vi "enthalpy of vaporization.vi"(8 "error in (no error)":errorcluster, 11 "TK":dbl) -> (0 "error out":errorcluster, 3 "function return":dbl)   [LabVIEW 2011, in "fsteam.lvlib"]
doc: "extern double enthalpy_of_vaporization(double TK);"
uses:
  <userlib>/fsteam/fsteam.lvlib
  <userlib>/fsteam/fsteam.dll
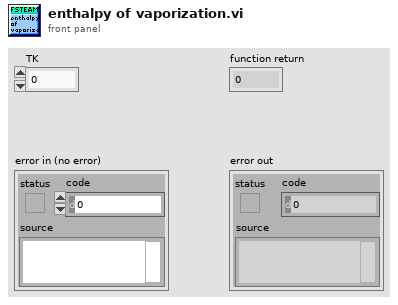
[diagram p1: front panel]
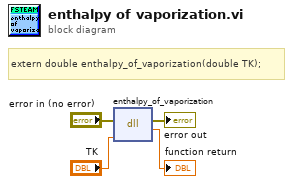
[diagram p0: block diagram]
diagram:
  # "extern double enthalpy_of_vaporization(double TK);"
  n1 = dll-call lib="C:/Program Files (x86)/National Instruments/LabVIEW 2011/user.lib/fsteam/fsteam.*" fn="enthalpy_of_vaporization"(error in="error in (no error)", "TK"="TK") -> (error out=→"error out":errorcluster, →"function return":dbl)  [unwired: 3 in, 1 out]
